vi "Move Cost.vi"(8 "Room Slot":i32, 9 "Destination Position":i32, 10 "Source Position":i32, 11 "Amphipod Type Index":i32) -> (3 "Move Cost":u64)   [LabVIEW 2019, in "23.lvlib"]
uses:
  23.lvlib
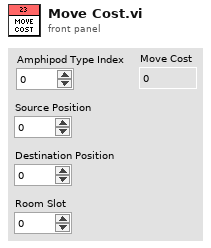
[diagram p1: front panel]
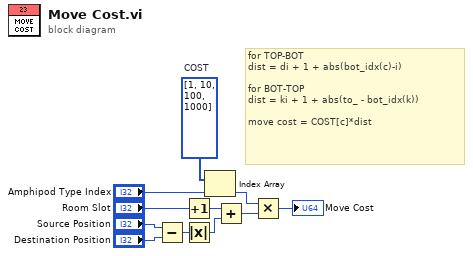
[diagram p0: block diagram]
diagram:
  w11 = u64[] [1, 10, 100, 1000]  # COST
  # "for TOP-BOT\ndist = di + 1 + abs(bot_idx(c)-i) \n\nfor BOT-TOP\ndist = ki + 1 + abs(to_ - bot_idx(k))\n\nmove cost = COST[c]*dist"
  n1 = Subtract(x="Source Position", y="Destination Position") -> (x-y=w2:i32)
  n2 = Increment(x="Room Slot") -> (x+1=w4:i32)
  n3 = Absolute Value(x=w2) -> (abs(x)=w3:i32)
  n4 = Index Array(array=w11, index="Amphipod Type Index") -> (element=w6:u64)
  n5 = Add(x=w4, y=w3) -> (x+y=w5:i32)
  n6 = Multiply(x=w6, y=w5) -> (x*y=→"Move Cost":u64)
